vi "g2Cal 160 MHz.vi"() -> ()   [LabVIEW 2015]
uses:
  <vilib>/Platform/TimedLoop/XDataNode/timing_clust.ctl
  <vilib>/Platform/TimedLoop/XDataNode/nitl_modes.ctl
  <vilib>/Platform/TimedLoop/XDataNode/wakeup.ctl
  <vilib>/rvi/Emulation/niFpgaGetClockAttributes.vi
  <vilib>/rvi/Emulation/niFpgaSctlEmulationGetInTimedLoop.vi
  <vilib>/rvi/Emulation/niFpgaEmulationReportErrorSimple.vi
  <vilib>/rvi/DataTransferAndStorage/Container/Common/niFpgaContainerGetUniqueNameForEmu.vi
  <vilib>/rvi/DataTransferAndStorage/Container/Common/niFpgaContainerSetEmuInfo.vi
  <vilib>/rvi/eio/common/nirviEmuReportErrorAndStop.vi
  <vilib>/rvi/Emulation/niFpgaCriticalErrorInLSC.vi
  Tick Count (U64) Global.vi
  <vilib>/rvi/DataTransferAndStorage/Container/Common/niFpgaContainerExecOnDevCompGetState.vi
  <vilib>/rvi/Emulation/niFpgaEmulationIsFPGAContextNoSignature.vi
  <vilib>/rvi/errors/niFpgaSetErrorForExecOnDevCompSimple.vi
  <vilib>/rvi/FIFO/Fifo_Resource/nirvififoEmulationSetSize.vi
  <vilib>/rvi/FIFO/Fifo_Resource/nirviFifoEmulationQueueMgr.vi
  <instcachedir>/0/nirviFifoEmulationQueueMgr_E5CAEC123FF24DC58D834DCA3CDAA9B5.lvgen/nirviFifoEmulationQueueMgr_E5CAEC123FF24DC58D834DCA3CDAA9B5_000.vi
  <vilib>/rvi/FIFO/Fifo_Resource/nirvififoEmulationDetermineInputValidOut.vi
  <vilib>/rvi/FIFO/Fifo_Resource/nirvififoEmulationCreateLock.vi
  <vilib>/rvi/Emulation/niFpgaProcessEmulError.vi
  <vilib>/rvi/FIFO/Fifo_Resource/nirvififoEmulationObtainLock.vi
  <vilib>/rvi/FIFO/Fifo_Resource/nirvififoEmulationReleaseLock.vi
  <vilib>/rvi/occurrence/nirviWaitOnOccurrenceBase.vi
  <vilib>/rvi/errors/nirviReportUnexpectedCaseInternalError.vi
  <vilib>/rvi/errors/nirviReportUnexpectedCaseInternalError (U32).vi
  <vilib>/Utility/error.llb/Clear Errors.vi
  <vilib>/rvi/interface/RandomDataEmulation/niFpgaRandomDataHandleErrors.vi
  <vilib>/rvi/eio/common/nirviEmuTemplateMethod_errors.vi
  <vilib>/Platform/TimedLoop/XDataNode/XDataNode.xnode
  <vilib>/rvi/LocalResourceManager/LocalResourceManager.xnode
  <vilib>/rvi/FXPMathLib/FxpMul/XNode/nifxpmath_Multiplier.xnode
  <vilib>/rvi/FXPMathLib/FxpSub/XNode/nifxpmath_Sub.xnode
  <vilib>/rvi/DataTransferAndStorage/Container/XNode/niFpgaContainer.xnode
  <vilib>/rvi/FIFO/Fifo_Resource/niFpgaFifoEmulationRefIn.vi
  <vilib>/eio/EIONode/EIONode.xnode
  <vilib>/rvi/interface/RandomDataEmulation/nirviRandomDataFpgaReadWriteTemplate.vi
  <vilib>/Platform/TimedLoop/XDataNode/XDNodeRunTimeDep.lvlib
  <vilib>/rvi/FXPMathLib/sim/FxpSim.dll
panel:
  in  "Frequency (MHz)":fxp<+,16,4>=0.00634765625
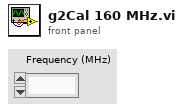
[diagram p1: front panel]
types:
  T1 = typedef "XDNodeRunTimeDep.lvlib/timing_clust.ctl" = cluster{"Expected End [f-1]":u64, "Actual End [f-1]":u64, "Finished Late? [f-1]":bool, "Expected End [i-1]":u64, "Actual End [i-1]":u64, "Finished Late? [i-1]":bool, "Expected Start [i]":u64, "Actual Start [i]":u64, "Expected Start [f]":u64, "Actual Start [f]":u64, "Source Name":string, "Structure Name":string, "Period":i64, "Deadline":i64, "Offset":i64, "Start":i64, "Priority":i32, "Timeout":i32, "Mode":T2, "Wakeup Reason":T3, "Error":errorcluster, "Source Type":string, "Secondary Source Type":string, "Global End Time":u64, "Global Start Time":u64, "Frame Duration":u64, "Iteration Duration":u64, "Assigned CPU":i32, "I/O Scan Engine Mode":u32}
  T2 = typedef "XDNodeRunTimeDep.lvlib/nitl_modes.ctl" = enum32{"No Change", "Process missed periods, maintain original phase", "Discard missed periods, maintain original phase", "Process missed periods, ignore original phase", "Discard missed periods, ignore original phase"}
  T3 = typedef "XDNodeRunTimeDep.lvlib/wakeup.ctl" = enum32{"Normal", "Aborted", "Asynchronous wakeup", "Timing source error", "Timed loop error", "Timeout"}
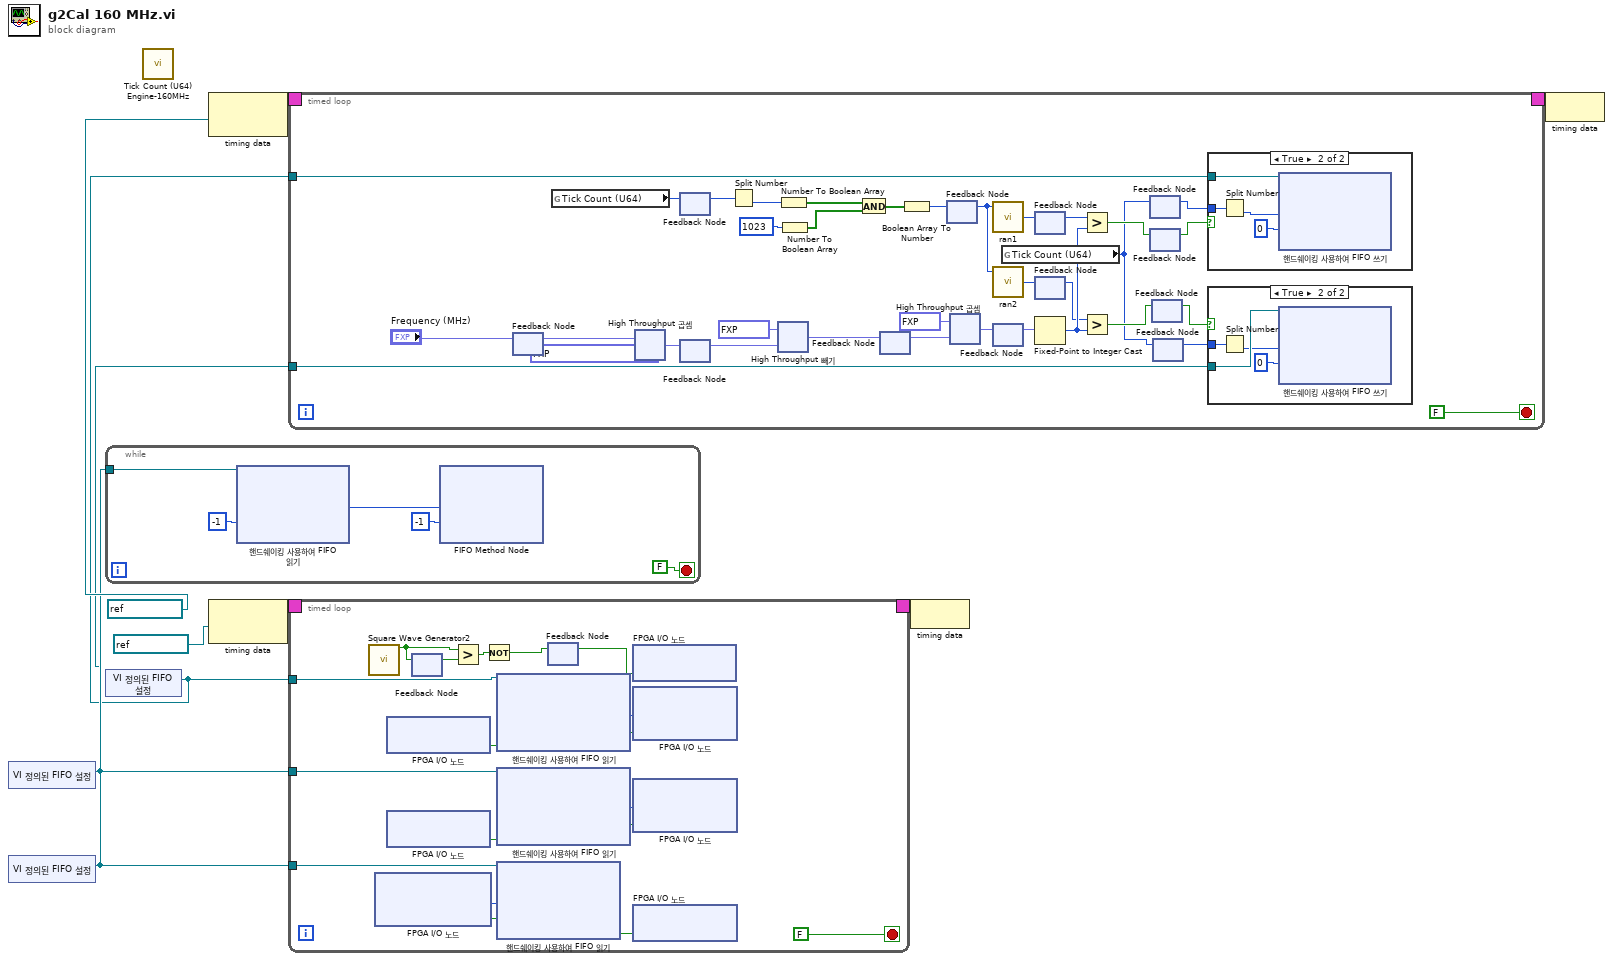
[diagram p0: block diagram]
diagram:
  n1 = xnode "VI 정의된 FIFO 설정"() -> ("FIFO Out"=w1:refnum<k21>)
  n2 = xnode "VI 정의된 FIFO 설정"() -> ("FIFO Out"=w3:refnum<k21>)
  n3 = while {
    tunnel: w3 -> [w14]
    stop <- FALSE stop-if-true
    n4 = xnode ("핸드쉐이킹 사용하여 FIFO 읽기")("Timeout"=-1 ("타임아웃"), "FIFO In"=w14) -> ("Element"=w12:u32)  [unwired: 2 out]
    n5 = xnode ("FIFO Method Node")("Element"=w12, "Timeout"=-1 ("타임아웃")) -> ()  [unwired: 1 in, 2 out]
  }
  n6 = xnode "VI 정의된 FIFO 설정"() -> ("FIFO Out"=w2:refnum<k21>)
  n7 = call "Tick Count (U64) Engine-160MHz.vi"() -> ()  [unwired: 1 out]
  n8 = node-c288(refnum<k21> "160MHz" ("소스 이름")) -> (w6:T1)
  n9 = node-c288(refnum<k21> "160MHz" ("소스 이름")) -> (w9:T1)
  n10 = timed-loop {
    timing: w6 -> [_]
    timing-out: [_] -> w5
    tunnel: w2 -> [w25]
    tunnel: w1 -> [w24]
    stop <- FALSE stop-if-true
    n11 = feedback #1() -> (w16:fxp<+,16,4>)  [unwired: 1 in]
    n12 = feedback-in #1("Frequency (MHz)") -> ()
    n13 = global read "Tick Count (U64) Global.vi" "Tick Count (U64)"() -> (w29:u64)
    n14 = xnode ("High Throughput 곱셈")("x"=w16, "y"=fxp<+,16,0> 0.0124969482421875) -> ("x*y"=w42:fxp<+,16,0>)
    n15 = feedback #2() -> (w28:u64)  [unwired: 1 in]
    n16 = feedback-in #2(w29) -> ()
    n17 = feedback #3() -> (w43:fxp<+,16,0>)  [unwired: 1 in]
    n18 = feedback-in #3(w42) -> ()
    n19 = Split Number(x=w28) -> (lo(x)=w27:u32)  [unwired: 1 out]
    n20 = xnode "High Throughput 빼기"("x"=fxp<+,16,0> 0.9999847412109375, "y"=w43) -> ("x-y"=w41:fxp<+,16,0>)
    n21 = Number To Boolean Array(number=w27) -> (Boolean array=w35:bool[])
    n22 = Number To Boolean Array(number=u32 1023 ("숫자")) -> (Boolean array=w34:bool[])
    n23 = And(x=w35, y=w34) -> (x .and. y?=w32:bool[])
    n24 = feedback #4() -> (w40:fxp<+,16,0>)  [unwired: 1 in]
    n25 = feedback-in #4(w41) -> ()
    n26 = Boolean Array To Number(Boolean array=w32) -> (number=w31:u32)
    n27 = feedback #5() -> (w30:u32)  [unwired: 1 in]
    n28 = feedback-in #5(w31) -> ()
    n29 = xnode ("High Throughput 곱셈")("x"=fxp<+,16,16> 32786.0, "y"=w40) -> ("x*y"=w45:fxp<+/-,16,16>)
    n30 = call "ran1"("address"=w30) -> ("data out"=w37:i16)  [unwired: 8 in]
    n31 = call "ran2"("address"=w30) -> ("data out"=w36:i16)  [unwired: 8 in]
    n32 = feedback #6() -> (w44:fxp<+/-,16,16>)  [unwired: 1 in]
    n33 = feedback-in #6(w45) -> ()
    n34 = global read "Tick Count (U64) Global.vi" "Tick Count (U64)"() -> (w17:u64)
    n35 = feedback #7() -> (w38:i16)  [unwired: 1 in]
    n36 = feedback-in #7(w37) -> ()
    n37 = feedback #8() -> (w39:i16)  [unwired: 1 in]
    n38 = feedback-in #8(w36) -> ()
    n39 = Fixed-Point to Integer Cast(1:w44) -> (0:w46:i16)
    n40 = Greater?(x=w38, y=w46) -> (0:w22:bool)
    n41 = Greater?(x=w39, y=w46) -> (0:w19:bool)
    n42 = feedback #9() -> (w23:u64)  [unwired: 1 in]
    n43 = feedback-in #9(w17) -> ()
    n44 = feedback #10() -> (w21:bool)  [unwired: 1 in]
    n45 = feedback-in #10(w22) -> ()
    n46 = feedback #11() -> (w20:bool)  [unwired: 1 in]
    n47 = feedback-in #11(w19) -> ()
    n48 = feedback #12() -> (w18:u64)  [unwired: 1 in]
    n49 = feedback-in #12(w17) -> ()
    n50 = case shown="True" w21 {
      tunnel: w25 -> [_ w57]
      tunnel: w23 -> [_ w55]
      frame False {
      }
      frame True {
        n51 = Split Number(x=w55) -> (lo(x)=w54:u32)  [unwired: 1 out]
        n52 = xnode ("핸드쉐이킹 사용하여 FIFO 쓰기")("Element"=w54, "Timeout"=0 ("타임아웃"), "FIFO In"=w57) -> ()  [unwired: 2 out]
      }
    }
    n53 = case shown="True" w20 {
      tunnel: w24 -> [_ w52]
      tunnel: w18 -> [_ w51]
      frame False {
      }
      frame True {
        n54 = Split Number(x=w51) -> (lo(x)=w50:u32)  [unwired: 1 out]
        n55 = xnode ("핸드쉐이킹 사용하여 FIFO 쓰기")("Element"=w50, "Timeout"=0 ("타임아웃"), "FIFO In"=w52) -> ()  [unwired: 2 out]
      }
    }
  }
  n56 = timed-loop {
    timing: w9 -> [_]
    timing-out: [_] -> w8
    tunnel: w2 -> [w77]
    tunnel: w1 -> [w76]
    tunnel: w3 -> [w65]
    stop <- FALSE stop-if-true
    n57 = call "Square Wave Generator2"() -> ("square wave out"=w74:bool)  [unwired: 15 in]
    n58 = xnode "FPGA I/O 노드"() -> ("g2Cal\\g2Dat"=w64:u32, "g2Cal\\g2V"=w63:bool)  [unwired: 2 in, 2 out]
    n59 = xnode "FPGA I/O 노드"() -> ("g2Cal\\a1R"=w71:bool)  [unwired: 1 in, 1 out]
    n60 = xnode "FPGA I/O 노드"() -> ("g2Cal\\a2R"=w66:bool)  [unwired: 1 in, 1 out]
    n61 = feedback #13() -> (w75:bool)  [unwired: 1 in]
    n62 = feedback-in #13(w74) -> ()
    n63 = Greater?(x=w74, y=w75) -> (0:w73:bool)
    n64 = Not(x=w73) -> (.not. x?=w61:bool)
    n65 = xnode ("핸드쉐이킹 사용하여 FIFO 읽기")("Ready for Output"=w71, "FIFO In"=w77) -> ("Element"=w70:u32, "Output Valid"=w69:bool)  [unwired: 1 out]
    n66 = xnode ("핸드쉐이킹 사용하여 FIFO 읽기")("Ready for Output"=w66, "FIFO In"=w76) -> ("Element"=w68:u32, "Output Valid"=w67:bool)  [unwired: 1 out]
    n67 = xnode ("핸드쉐이킹 사용하여 FIFO 읽기")("Element"=w64, "Input Valid"=w63, "FIFO In"=w65) -> ("Ready for Input"=w62:bool)  [unwired: 1 out]
    n68 = feedback #14() -> (w60:bool)  [unwired: 1 in]
    n69 = feedback-in #14(w61) -> ()
    n70 = xnode "FPGA I/O 노드"("g2Cal\\RST"=w60) -> ()  [unwired: 1 in, 1 out]
    n71 = xnode "FPGA I/O 노드"("g2Cal\\a1"=w70, "g2Cal\\a1V"=w69) -> ()  [unwired: 2 in, 2 out]
    n72 = xnode "FPGA I/O 노드"("g2Cal\\a2"=w68, "g2Cal\\a2V"=w67) -> ()  [unwired: 2 in, 2 out]
    n73 = xnode "FPGA I/O 노드"("g2Cal\\g2R"=w62) -> ()  [unwired: 1 in, 1 out]
  }
  n74 = node-c288(w8) -> ()
  n75 = node-c288(w5) -> ()
